vi "globalVariables.vi"() -> ()   [LabVIEW 2012]
uses:
  TimeValue.ctl
  SensorSettingCtl.ctl
panel:
  out "globalAccessSemaphore":T1
  in  "MaxNrOfSamples":i32=1000000
  in  "Path for measuring results":path
  out "Program running":bool[](array[boolean])
  in  "stop measurement":bool
  out "Saved Configuration":T2[](array[typedef])
  in  "AllValues":T3[][](array[typedef])
  in  "NewestValues":T3[](array[typedef])
  out "Errors":errorcluster[](array[cluster])
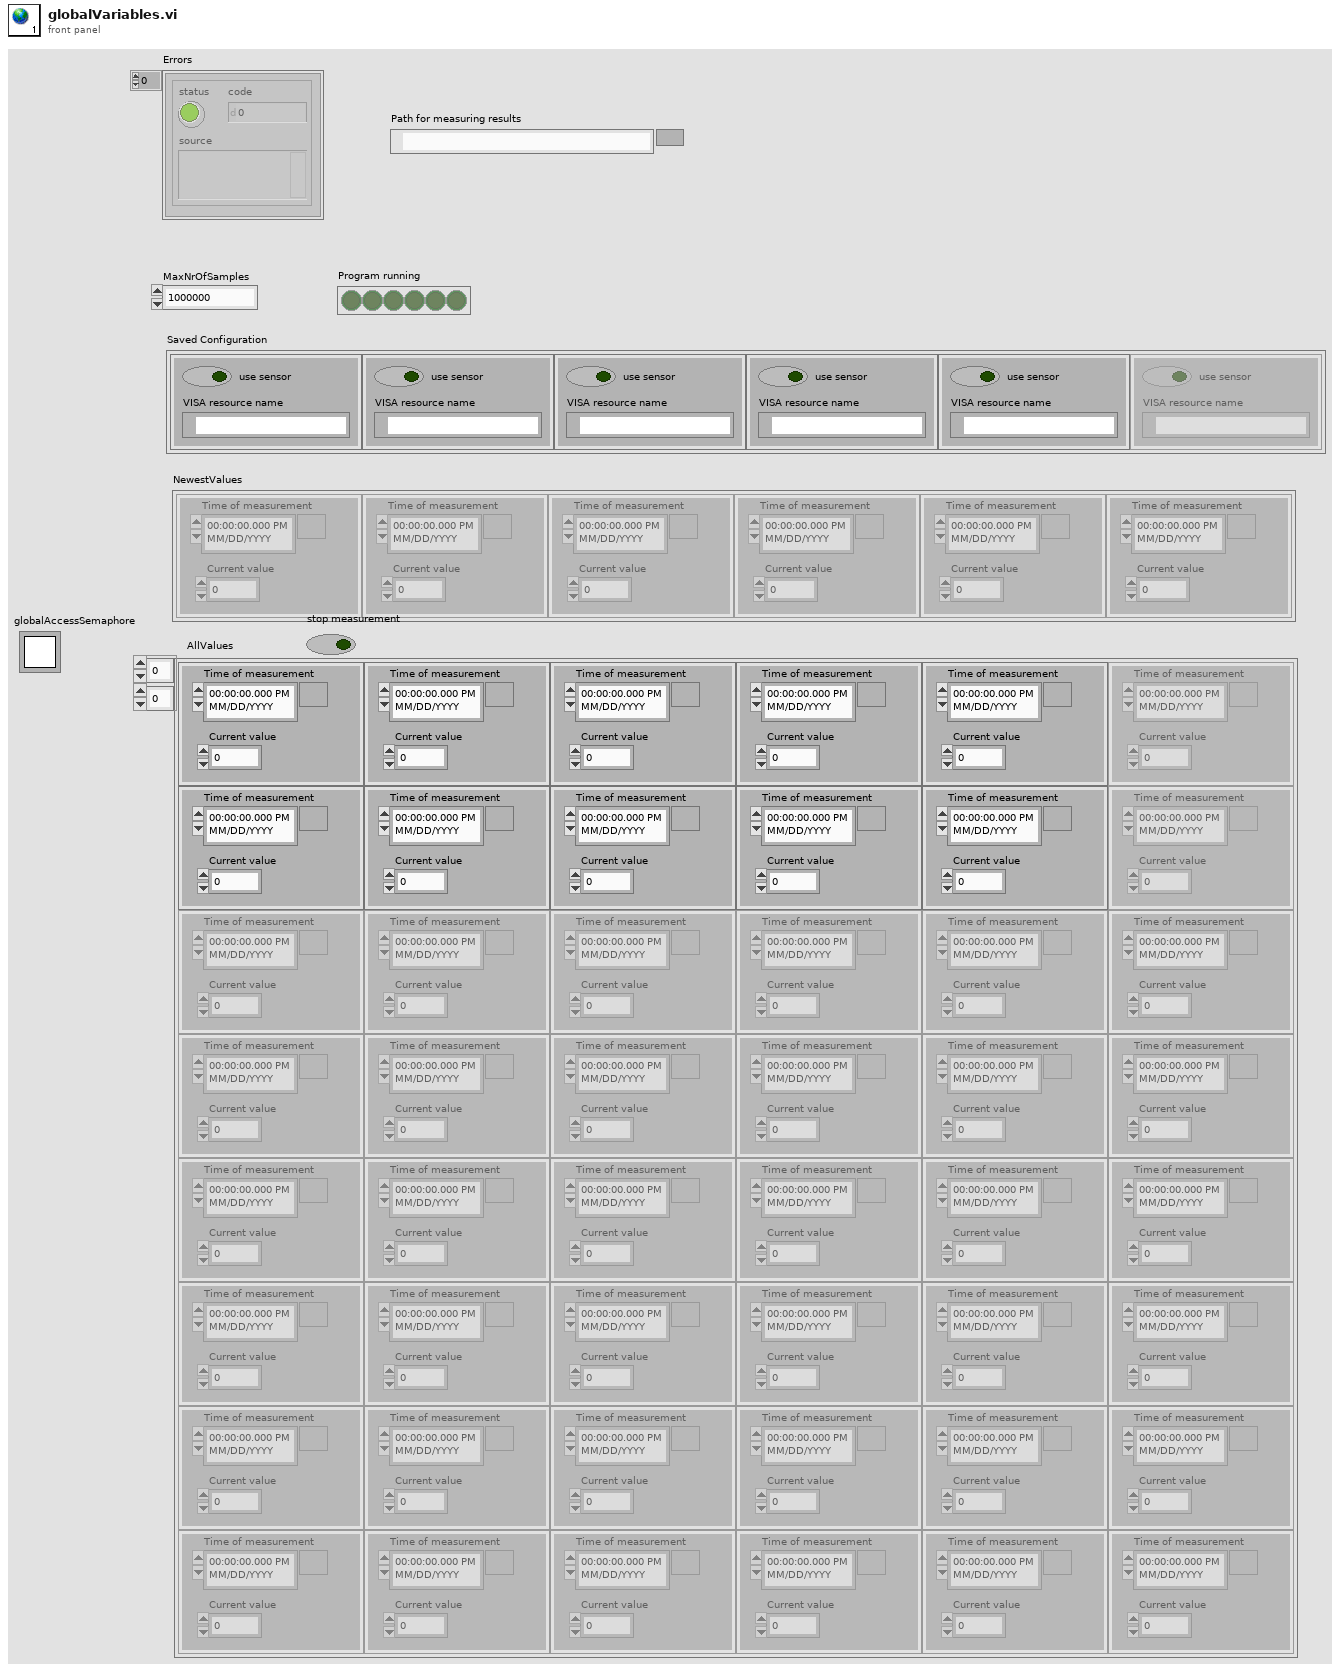
[diagram p1: front panel]
types:
  T1 = typedef "Semaphore RefNum" = refnum<k1>
  T2 = typedef "SensorSettingCtl.ctl" = cluster{"VISA resource name":refnum<visa-resource-name>, "use sensor":bool}
  T3 = typedef "TimeValue.ctl" = cluster{"Time of measurement":timestamp, "Current value":dbl}
diagram:
